vi "Fault ID Setup.vi"(0 "LBCB Number":T3) -> (1 "Act Inc Setup":T1, 2 "Cart Inc Setup":T1, 3 "Actuator Displacement Setup":T1, 4 "Actuator Force Setup":T1, 5 "Cartesian Disp Setup":T1, 6 "Cartesian Force Setup":T1)   [LabVIEW 2013]
uses:
  Data Access Objects/Metadata/LBCB Number.ctl
  Fault Id.ctl
  Fault Type.ctl
  Space Type.ctl
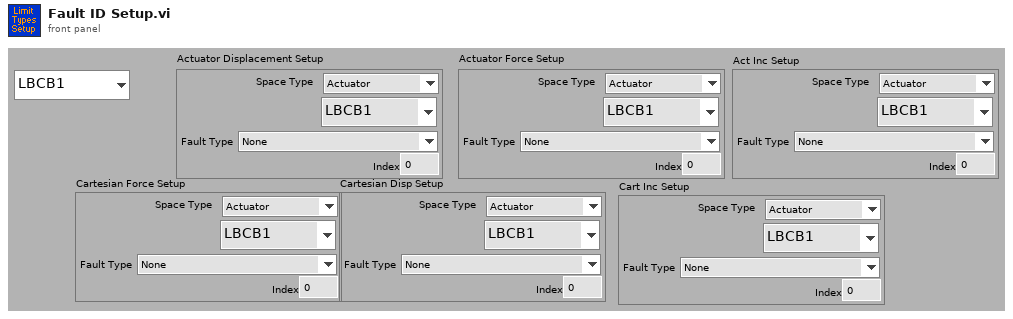
[diagram p1: front panel]
types:
  T1 = typedef "Fault Id.ctl" = cluster{"Fault Type":T2, "LBCB Number":T3, "Index":u32, "Space Type":T4}
  T2 = typedef "Fault Type.ctl" = enum16{"None", "Command", "Displacement", "Force", "Increment"}
  T3 = typedef "LBCB Number.ctl" = enum16{"LBCB1", "LBCB2"}
  T4 = typedef "Space Type.ctl" = enum16{"Actuator", "Cartesian"}
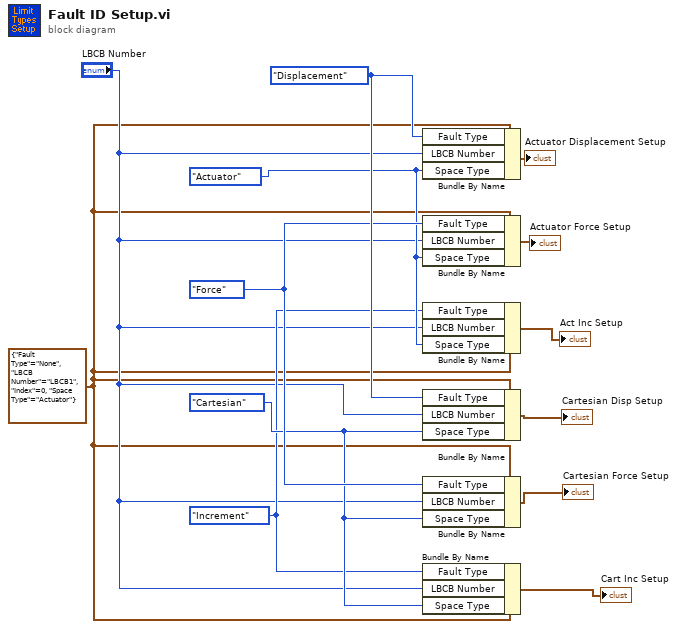
[diagram p0: block diagram]
diagram:
  w3 = Fault_Type."Increment" ("Fault Type")
  w6 = Space_Type."Cartesian" ("Space Type")
  w10 = Fault_Type."Force" ("Fault Type")
  w4 = Space_Type."Actuator" ("Space Type")
  w11 = Fault_Type."Displacement" ("Fault Type")
  w1 = T1 {"Fault Type"=enum."None", "LBCB Number"=enum."LBCB1", "Index"=0, "Space Type"=enum."Actuator"} ("Fault Id In")
  n1 = Bundle By Name(cluster=w1, "Fault Type"=w11, "LBCB Number"="LBCB Number", "Space Type"=w4) -> (→"Actuator Displacement Setup":T1)
  n2 = Bundle By Name(cluster=w1, "Fault Type"=w10, "LBCB Number"="LBCB Number", "Space Type"=w4) -> (→"Actuator Force Setup":T1)
  n3 = Bundle By Name(cluster=w1, "Fault Type"=w3, "LBCB Number"="LBCB Number", "Space Type"=w4) -> (→"Act Inc Setup":T1)
  n4 = Bundle By Name(cluster=w1, "Fault Type"=w11, "LBCB Number"="LBCB Number", "Space Type"=w6) -> (→"Cartesian Disp Setup":T1)
  n5 = Bundle By Name(cluster=w1, "Fault Type"=w10, "LBCB Number"="LBCB Number", "Space Type"=w6) -> (→"Cartesian Force Setup":T1)
  n6 = Bundle By Name(cluster=w1, "Fault Type"=w3, "LBCB Number"="LBCB Number", "Space Type"=w6) -> (→"Cart Inc Setup":T1)
